vi "CMN_Parse Arithmetic Expression.vi"(1 "Arithmetic Expression":string="1 + 3.1415 * 2*2") -> (0 "Result":dbl format="%.6f")   [LabVIEW 2016]
doc: "This somewhat more advanced example VI shows how to use the Scan String for Tokens and Scan From String primitives to write an infix arithmetic expression parser."
panel:
  # "Arithmetic expression (infix) parser"
  # "Enter an arithmetic expression into the control below.  Known operators are: +, -, *, /, %, (, )\nPress <ctrl-h> for more information."
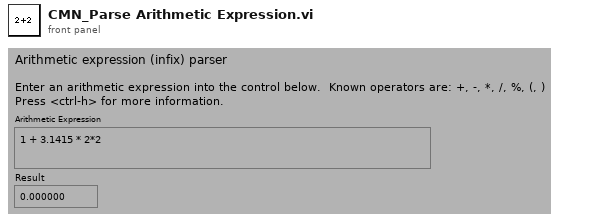
[diagram p1: front panel]
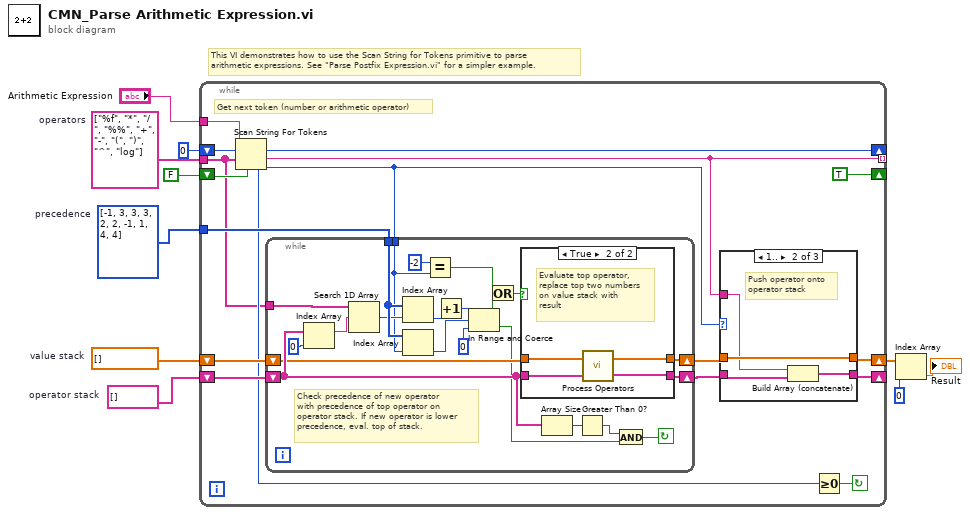
[diagram p0: block diagram]
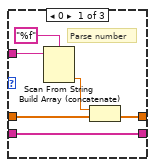
[diagram p3: hidden frame]
diagram:
  w2 = i32[] [-1, 3, 3, 3, 2, 2, -1, 1, 4, 4]  # precedence
  w6 = string[] ["%f", "*", "/", "%%", "+", "-", "(", ")", "^", "log"]  # operators
  w7 = string[] []  # operator stack
  w8 = dbl[] []  # value stack
  # "This VI demonstrates how to use the Scan String for Tokens primitive to parse\narithmetic expressions. See \"Parse Postfix Expression.vi\" for a simpler example."
  n1 = while {
    tunnel: w2 -> [w20]
    shift-left: w7 -> [w17]
    shift-right: [w18] -> _
    shift-left: w8 -> [w15]
    shift-right: [w19] -> w5
    tunnel: [w11] -> _ mode=indexing
    tunnel: w6 -> [w12]
    tunnel: "Arithmetic Expression" -> [w22]
    shift-left: FALSE ("use cached delim/oper data? (F)") -> [w24]
    shift-right: [TRUE ("use cached delim/oper data? (F)")] -> _
    shift-left: 0 ("offset past token") -> [w23]
    shift-right: [w26] -> _
    stop <- w21 continue-if-true
    # "Get next token (number or arithmetic operator)"
    n2 = Scan String For Tokens(4:w24, 7:w12, 8:w23, 9:w22) -> (0:w13:i32, 1:w11:string, 2:w26:i32)  [unwired: 3 out]
    n3 = while {
      shift-left: w15 -> [w35]
      shift-right: [w34] -> w14
      shift-left: w17 -> [w39]
      shift-right: [w40] -> w16
      tunnel: w13 -> [w31]
      tunnel: w20 -> [w41]
      tunnel: w12 -> [w46]
      stop <- w37 continue-if-true
      # "Check precedence of new operator\nwith precedence of top operator on\noperator stack. If new operator is lower\nprecedence, eval. top of stack."
      n4 = Index Array(array=w39, index=0) -> (element=w45:string)
      n5 = Search 1D Array(1D array=w46, element=w45) -> (index of element=w32:i32)  [unwired: 1 out]
      n6 = Index Array(array=w41, index=w32) -> (element=w30:i32)
      n7 = Index Array(array=w41, index=w31) -> (element=w29:i32)
      n8 = Equal?(x=-2, y=w31) -> (x = y?=w43:bool)
      n9 = Increment(x=w30) -> (x+1=w28:i32)
      n10 = In Range and Coerce(upper limit=w28, x=w29, lower limit=0 ("x")) -> (In Range?=w33:bool)  [unwired: 1 out]
      n11 = Or(x=w43, y=w33) -> (x .or. y?=w42:bool)
      n12 = case shown="True" w42 {
        tunnel: [w49 w51] -> w34
        tunnel: w35 -> [w49 w53]
        tunnel: w39 -> [w48 w52]
        tunnel: [w48 w50] -> w40
        frame False {
        }
        frame True {
          # "Evaluate top operator, \nreplace top two numbers\non value stack with \nresult"
          n13 = call "Process Operators.vi"("opers in"=w52, "values in"=w53) -> ("opers out"=w50:string[], "values out"=w51:dbl[])
        }
      }
      n14 = Array Size(array=w39) -> (size(s)=w36:i32)
      n15 = Greater Than 0?(x=w36) -> (x > 0?=w38:bool)
      n16 = And(x=w38, y=w33) -> (x .and. y?=w37:bool)
    }
    n17 = case shown="1.." w13 {
      tunnel: w11 -> [w59 w61 _]
      tunnel: w14 -> [w55 w63 w65]
      tunnel: [w58 w63 w65] -> w19
      tunnel: w16 -> [w56 w60 w64]
      tunnel: [w56 w62 w64] -> w18
      frame 0 {
        # "Parse number"
        n18 = Scan From String(format string="%f", input string=w59) -> (output 1=w54:dbl)  [unwired: 2 in, 4 out]
        n19 = Build Array (concatenate)(w54, w55) -> (w58:dbl[])
      }
      frame 1.. {
        # "Push operator onto\noperator stack"
        n20 = Build Array (concatenate)(w61, w60) -> (w62:string[])
      }
      frame Default {
        # "Illegal input or end of \nstring, do nothing"
      }
    }
    n21 = Greater Or Equal To 0?(x=w13) -> (x >= 0?=w21:bool)
  }
  n22 = Index Array(array=w5, index=0) -> (element=→"Result":dbl)
